vi "svfa_Average Array (complex) No State_spectrum state.vi"(6 "previous avg complex spectrum":T3 {"complex array" format="%.2f"; "df" format="%.2f"; "f0" format="%.2f"}, 7 "processing control":T1(ring), 8 "averages completed in":dbl format="%.2f", 9 "averaging parameters":T2={"averaging mode"=enum."No averaging", "weighting mode"=enum."Linear", "number of averages"=10, "linear mode"=enum."Auto restart"}, 11 "array":cdb[](array[numeric]) format="%.2f") -> (0 "averages completed out":dbl, 1 "averaging done":bool, 4 "avg complex spectrum":T3 {"complex array" format="%.2f"; "df" format="%.2f"; "f0" format="%.2f"})   [LabVIEW 2017]
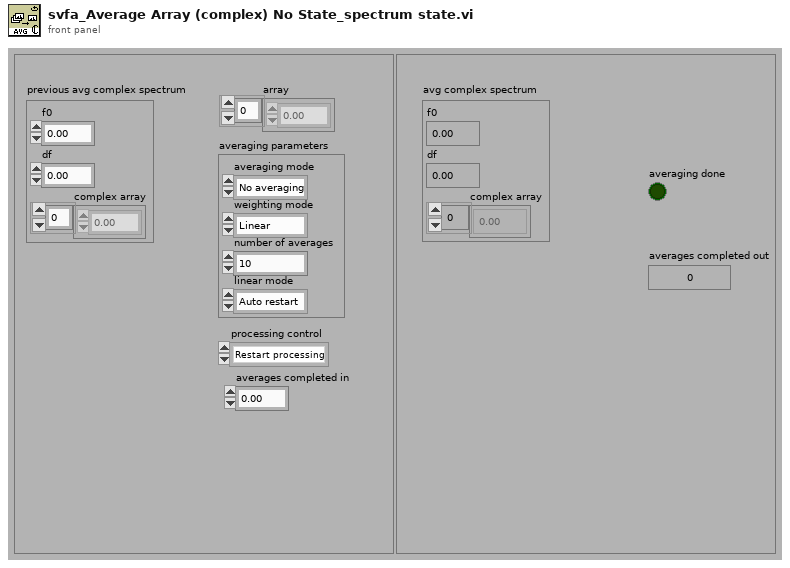
[diagram p1: front panel]
types:
  T1 = enum16{"Restart processing", "Continue processing", "Skip processing"}
  T2 = cluster{"averaging mode":enum16{"No averaging", "Vector averaging", "RMS averaging", "Peak hold"}, "weighting mode":enum16{"Linear", "Exponential"}, "number of averages":u32, "linear mode":enum16{"One shot", "Auto restart"}}
  T3 = cluster{"f0":dbl, "df":dbl, "complex array":cdb[]}
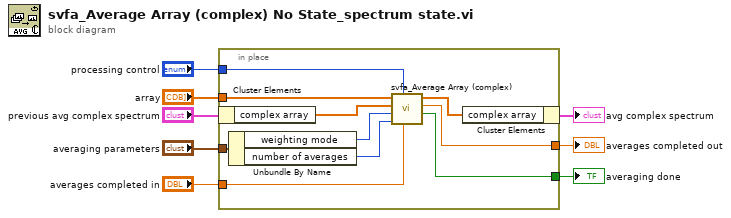
[diagram p0: block diagram]
diagram:
  n1 = in-place {
    in-place-border: [w18] -> w8
    in-place-border: "array" -> [w17]
    in-place-border: [w16] -> w6
    in-place-border: "processing control" -> [w15]
    in-place-border: "averages completed in" -> [w14]
    in-place-border: "averaging parameters" -> [w11]
    n2 = in-place-cluster #1("previous avg complex spectrum") -> ("complex array"=w13:cdb[])
    n3 = Unbundle By Name(w11) -> ("weighting mode"=w10:enum16{"Linear", "Exponential"}, "number of averages"=w9:u32)
    n4 = call <vilib>:"svfa_Average Array (complex).vi"("averages completed in"=w14, "processing control"=w15, "number of averages"=w9, "weighting mode"=w10, "previous average array"=w13, "array"=w17) -> ("averaging done"=w16:bool, "averages completed out"=w18:dbl, "average array"=w12:cdb[])  [unwired: 3 in]
    n5 = in-place-cluster #1("complex array"=w12) -> (→"avg complex spectrum":T3)
  }
  "averages completed out" <- w8
  "averaging done" <- w6
